vi "Read Block Length.vi"(8 "error in (no error)":errorcluster, 11 "Refnum in":refnum<k21>) -> (0 "error out":errorcluster, 1 "Block Size":u16, 2 "Array":string[](array[string]), 3 "data":T1[](array[typedef]) {"payload" format="%x"; "timestamp" format="%<%.7X\n%x>T"; "type" items=["CAN Data"=0, "CAN Remote"=1, "CAN Bus Error"=2, "CAN 2.0 Data"=8, "CAN FD Data"=16, "CAN FD+BRS Data"=24, "J1939 Data"=192, "Delay"=224, "Log Trigger"=225, "Start Trigger"=226]; "identifier" format="%x"}, 5 "Flow Control?":bool)   [LabVIEW 2014]
uses:
  <vilib>/xnet/xnet.llb/XNET Frame CAN.ctl
  <vilib>/xnet/xnet.llb/XNET Frame Type CAN.ctl
  <vilib>/xnet/xnet.llb/XNET Read (Frame CAN).vi
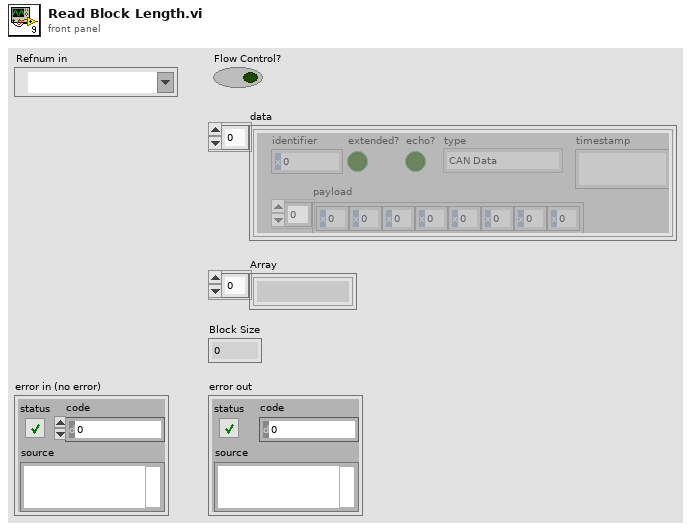
[diagram p1: front panel]
types:
  T1 = typedef "XNET Frame CAN.ctl" = cluster{"timestamp":timestamp, "payload":u8[], "identifier":u32, "type":T2, "extended?":bool, "echo?":bool}
  T2 = typedef "XNET Frame Type CAN.ctl" = u8
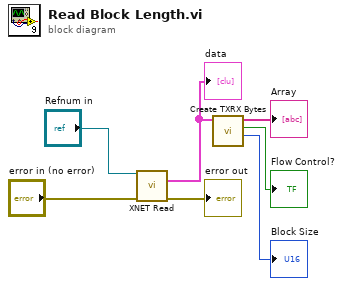
[diagram p0: block diagram]
diagram:
  n1 = call-poly <vilib>:"XNET Read.vi"("session in"="Refnum in", "error in (no error)"="error in (no error)") -> ("data"=w2:T1[], "error out"=→"error out":errorcluster)  [unwired: 10 in, 2 out]
  "data" <- w2
  n2 = call "Create TXRX Bytes.vi"("Cluster Array in"=w2) -> ("Array"=→"Array":string[], "Flow Control?"=→"Flow Control?":bool, "Block Size"=→"Block Size":u16)  [unwired: 7 in]
